vi "Write TDMS.vi"(4 "Append? [F]":bool, 6 "Igor Commands":string, 7 "path":path, 8 "error in (no error)":errorcluster, 9 "Comments":string, 10 "Data (Dictionary)":T1[](array[typedef]), 11 "LVtoITX in":refnum<class "LV to ITX.lvclass">) -> (0 "error out":errorcluster, 2 "path 2":path, 3 "LVtoITX out":refnum<class "LV to ITX.lvclass">)   [LabVIEW 2016, in "LV to ITX.lvclass"]
uses:
  LV to ITX.lvclass
  Typedefs/Dictionary--cluster.ctl
  Typedefs/Filetype--enum.ctl
  LV to ITX.lvclass/LV to ITX.ctl
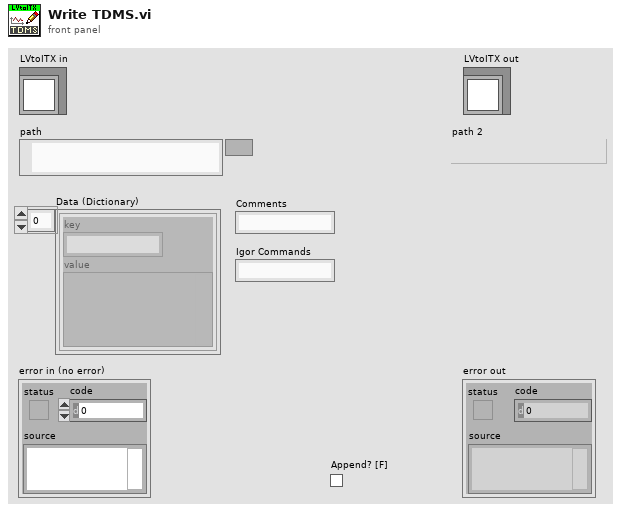
[diagram p1: front panel]
types:
  T1 = typedef "LV to ITX.lvclass/Dictionary--cluster.ctl" = cluster{"key":string, "value":variant}
  T2 = typedef "LV to ITX.lvclass/Filetype--enum.ctl" = enum16{"DAT", "ITX", "HDF5", "TDMS", "VI"}
  T3 = enum16{"open", "open or create", "create or replace", "create", "open (read-only)"}
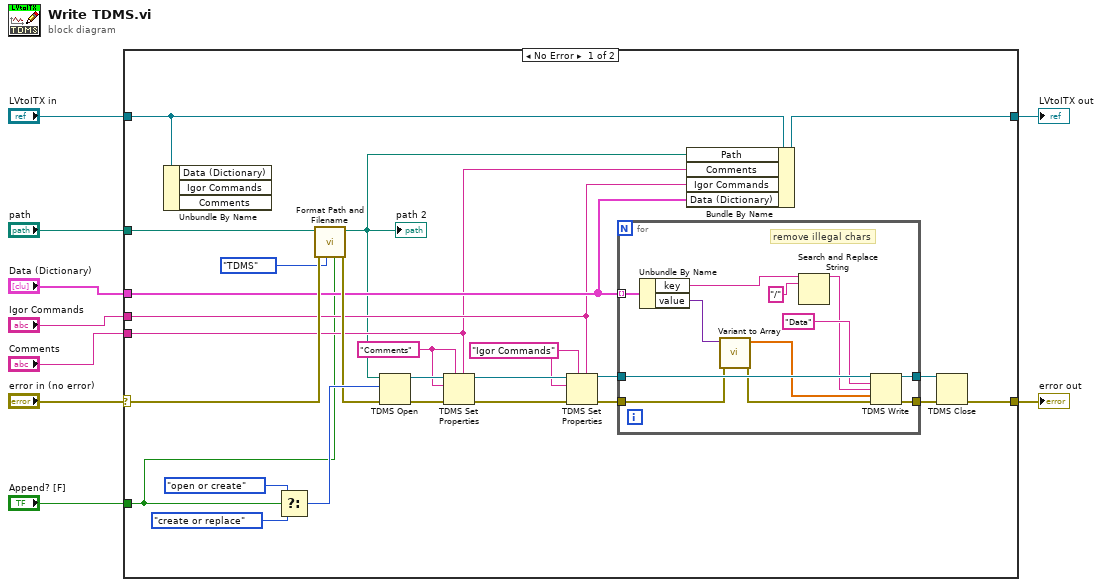
[diagram p0: block diagram]
diagram:
  n1 = case shown="No Error" "error in (no error)" {
    selector: "error in (no error)" -> [w20 w47]
    tunnel: [w27 w47] -> w6
    tunnel: [w15 w48] -> w7
    tunnel: "LVtoITX in" -> [w16 w48]
    tunnel: "Append? [F]" -> [w11 _]
    tunnel: "path" -> [w18 _]
    tunnel: "Comments" -> [w12 _]
    tunnel: "Igor Commands" -> [w13 _]
    tunnel: "Data (Dictionary)" -> [w14 _]
    frame No Error {
      w25 = "Igor Commands" ("attrib name")
      w24 = "Comments" ("attrib name")
      n2 = Unbundle By Name(w16) -> ()  [unwired: 3 out]
      n3 = Select(t=T3."open or create" ("operation (0:open)"), s=w11, f=T3."create or replace" ("operation (0:open)")) -> (s? t:f=w21:T3)
      n4 = call "Format Path and Filename.vi"("append? (F)"=w11, "Type (TDMS)"=Filetype--enum."TDMS", "error in"=w20, "path"=w18) -> ("error out"=w19:errorcluster, "path"=w10:path)  [unwired: 5 in, 1 out]
      "path 2" <- w10
      n5 = TDMS Open(8:w19, 10:w21, 11:w10) -> (0:w34:errorcluster, 3:w33:refnum<k34>)  [unwired: 4 in]
      n6 = TDMS Set Properties(5:w12, 7:w24, 8:w34, 10:w24, 11:w33) -> (0:w31:errorcluster, 3:w32:refnum<k34>)  [unwired: 1 in, 2 out]
      n7 = TDMS Set Properties(5:w13, 7:w25, 8:w31, 10:w25, 11:w32) -> (0:w30:errorcluster, 3:w29:refnum<k34>)  [unwired: 1 in, 2 out]
      n8 = for {
        tunnel: w14 -> [w40] mode=indexing
        tunnel: w30 -> [w37]
        tunnel: w29 -> [w45]
        tunnel: [w44] -> w28
        tunnel: [w43] -> w26
        # "remove illegal chars"
        n9 = Unbundle By Name(w40) -> ("key"=w41:string, "value"=w36:variant)
        n10 = call "Variant to Array.vi"("error in (no error)"=w37, "value"=w36) -> ("error out"=w38:errorcluster, "Array"=w35:dbl[])  [unwired: 8 in]
        n11 = Search and Replace String(input string=w41, search string="/") -> (result string=w39:string)  [unwired: 6 in, 3 out]
        n12 = TDMS Write(0:w45, 5:"Data" ("group name in (Untitled)"), 7:w39, 9:w35, 11:w38) -> (4:w43:refnum<k34>, 15:w44:errorcluster)  [unwired: 1 in, 2 out]
      }
      n13 = Bundle By Name(cluster=w16, "Path"=w10, "Comments"=w12, "Igor Commands"=w13, "Data (Dictionary)"=w14) -> (w15:refnum<class "LV to ITX.lvclass">)
      n14 = TDMS Close(8:w28, 11:w26) -> (0:w27:errorcluster)  [unwired: 1 out]
    }
    frame Error {
    }
  }
  "error out" <- w6
  "LVtoITX out" <- w7
